vi "Dequeue.vi"(8 "Error In":errorcluster, 9 "timeout (ms) (Default = -1)":i32=-1) -> (0 "Error Out":errorcluster, 2 "Data":variant, 3 "Command":T1)   [LabVIEW 2016, in "Error Manager.lvlib" / "Error Window Loop Queue.lvclass"]
doc: "Receives a command and feeds it to the module Message Handling Loop (MHL)."
uses:
  Error Window Loop Queue.lvclass
  Command (enum).ctl
  Queue Reference (library variable).vi
panel:
  # "Input\nInputs to the VI"
  # "Development\nControls or indicators that are useful for development or testing, but which are not outputs of the VI."
  # "Output\nOutputs of the VI"
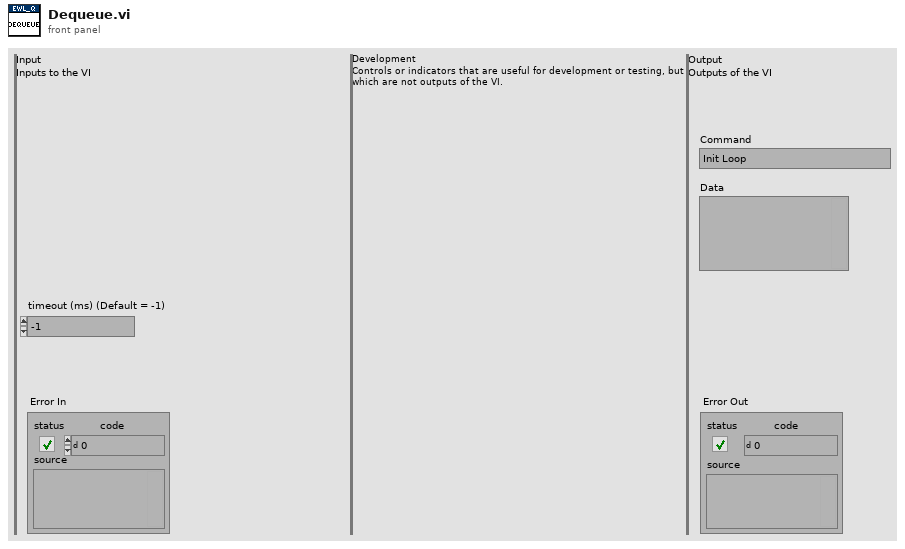
[diagram p1: front panel]
types:
  T1 = typedef "Error Manager.lvlib/Error Window Loop Queue.lvclass/Command (enum).ctl" = enum16{"Init Loop", "Close Loop", "Show Error Window"}
  T2 = typedef "Error Manager.lvlib/New Error Window Loop Queue.lvclass/Message (cluster).ctl" = cluster{"Command":T3, "Data":variant}
  T3 = typedef "Error Manager.lvlib/New Error Window Loop Queue.lvclass/Command (enum).ctl" = enum16{"Init Loop", "Close Loop", "Show Error Window"}
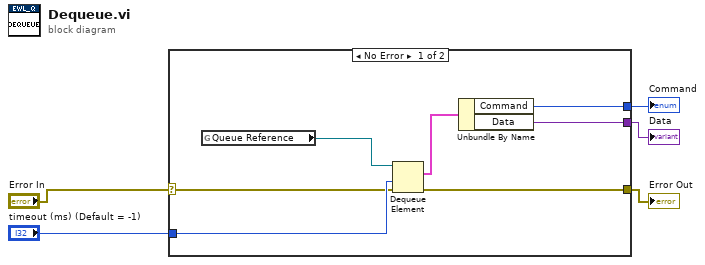
[diagram p0: block diagram]
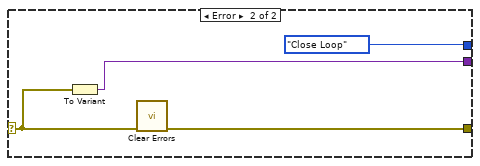
[diagram p2: hidden frame]
diagram:
  n1 = case shown="No Error" "Error In" {
    selector: "Error In" -> [w9 w15]
    tunnel: [w12 w14] -> w5
    tunnel: "timeout (ms) (Default = -1)" -> [w11 _]
    tunnel: [w10 w16] -> w3
    tunnel: [w6 Command_(enum)."Close Loop" ("Command")] -> w1
    frame No Error {
      n2 = global read "Queue Reference (library variable).vi" "Queue Reference"() -> (w7:refnum<queue>)
      n3 = Dequeue Element(queue=w7, timeout in ms (-1)=w11, error in (no error)=w9) -> (element=w8:T2, error out=w12:errorcluster)  [unwired: 2 out]
      n4 = Unbundle By Name(w8) -> ("Command"=w6:T3, "Data"=w10:variant)
    }
    frame Error {
      n5 = To Variant(anything=w15) -> (Variant=w16:variant)
      n6 = call <vilib>:"Clear Errors.vi"("error in (no error)"=w15) -> ("error out"=w14:errorcluster)  [unwired: 5 in, 1 out]
    }
  }
  "Error Out" <- w5
  "Command" <- w1
  "Data" <- w3
